vi "XL320_Checksum.vi"(1 "Input String":string) -> (0 "Checksum String":string)   [LabVIEW 2017, in "Dynamixel XL320.lvlib"]
doc: "Computes the checksum for the serial message."
uses:
  <instrlib>/Dynamixel XL320 (Drivers instrument)/Dynamixel XL320.lvlib
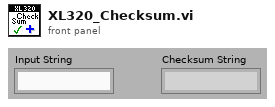
[diagram p1: front panel]
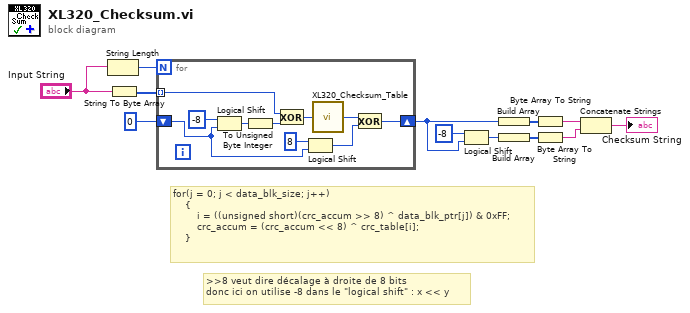
[diagram p0: block diagram]
diagram:
  # ">>8 veut dire décalage à droite de 8 bits\ndonc ici on utilise -8 dans le \"logical shift\" : x << y"
  # "for(j = 0; j < data_blk_size; j++)\n    {\n        i = ((unsigned short)(crc_accum >> 8) ^ data_blk_ptr[j]) & 0xFF;\n        crc_accum = (crc_accum << 8) ^ crc_table[i];\n    }"
  n1 = String Length(string="Input String") -> (length=w12:i32)
  n2 = String To Byte Array(string="Input String") -> (unsigned byte array=w10:u8[])
  n3 = for {
    N: w12 -> [_]
    tunnel: w10 -> [w18] mode=indexing
    shift-right: [w21] -> w2
    shift-left: u16 0 -> [w14]
    n4 = Logical Shift(y=i16 -8, x=w14) -> (x << y=w17:u16)
    n5 = To Unsigned Byte Integer(number=w17) -> (unsigned 8bit integer=w16:u8)
    n6 = Exclusive Or(1:w16, 2:w18) -> (0:w15:u8)
    n7 = Logical Shift(y=i16 8, x=w14) -> (x << y=w13:u16)
    n8 = call <instrlib>:"XL320_Checksum_Table.vi"("Numeric"=w15) -> ("Numeric 2"=w20:u16)
    n9 = Exclusive Or(1:w13, 2:w20) -> (0:w21:u16)
  }
  n10 = Logical Shift(y=i16 -8, x=w2) -> (x << y=w3:u16)
  n11 = Build Array(w2) -> (w8:u16[])
  n12 = Build Array(w3) -> (w5:u16[])
  n13 = Byte Array To String(unsigned byte array=w8) -> (string=w7:string)
  n14 = Byte Array To String(unsigned byte array=w5) -> (string=w4:string)
  n15 = Concatenate Strings(w7, w4) -> (→"Checksum String":string)
